vi "Mosbus_Master.vi"() -> ()   [LabVIEW 2020]
uses:
  <vilib>/NI/Modbus Library/API/Wrapper/Create TCP Master.vi
  <vilib>/ErrorRing/Error Ring.xnode
  <vilib>/NI/Modbus Library/API/Master/Modbus Master.lvclass
  <vilib>/NI/Modbus Library/API/Wrapper/API Main.lvlib
panel:
  in  "Thermometer":u16(slide) scale=0.0..100.0
  in  "Array 2":u16[](array[slide]) scale=0.0..100.0
  in  "Boolean 4":bool
  in  "Boolean 3":bool
  in  "Boolean 2":bool
  in  "Boolean":bool
  in  "stop":bool
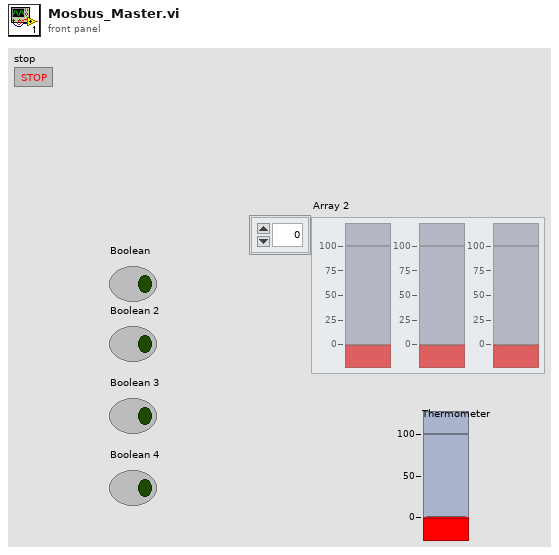
[diagram p1: front panel]
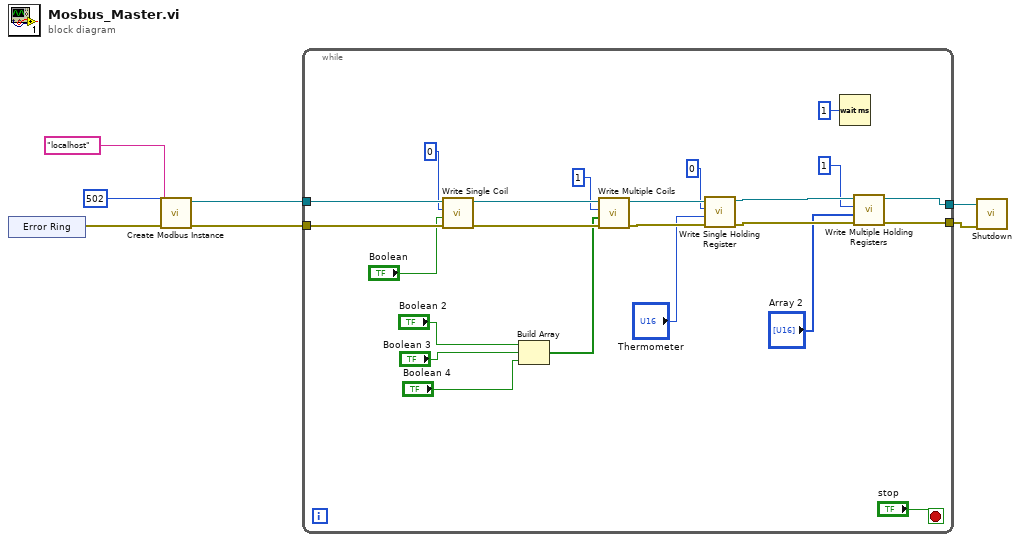
[diagram p0: block diagram]
diagram:
  n1 = xnode "Error Ring"() -> ("error out"=w5:errorcluster)
  n2 = call-poly <vilib>:"Create Modbus Instance.vi"("error in"=w5, "port (502)"=u16 502, "address"="localhost") -> ("error out"=w3:errorcluster, "TCP master instance"=w4:refnum<class "Modbus Master.lvclass">)  [unwired: 7 in]
  n3 = while {
    tunnel: w4 -> [w29]
    tunnel: w3 -> [w28]
    tunnel: [w13] -> w2
    tunnel: [w12] -> w1
    stop <- "stop" stop-if-true
    n4 = call-dynamic "Write Single Coil.vi"("error in"=w28, "coil to write"="Boolean", "address"=u16 0, "Modbus master in"=w29) -> ("error out"=w21:errorcluster, "Modbus master out"=w22:refnum<class "Modbus Master.lvclass">)  [unwired: 6 in]
    n5 = Build Array("Boolean 2", "Boolean 3", "Boolean 4") -> (w20:bool[])
    n6 = call-dynamic "Write Multiple Coils.vi"("error in"=w21, "coils to write"=w20, "starting address"=u16 1, "Modbus master in"=w22) -> ("error out"=w16:errorcluster, "Modbus master out"=w17:refnum<class "Modbus Master.lvclass">)  [unwired: 6 in]
    n7 = call-dynamic "Write Single Holding Register.vi"("error in"=w16, "register to write"="Thermometer", "address"=u16 0, "Modbus master in"=w17) -> ("error out"=w14:errorcluster, "Modbus master out"=w15:refnum<class "Modbus Master.lvclass">)  [unwired: 6 in]
    n8 = Wait (ms)(milliseconds to wait=u32 1) -> ()  [unwired: 1 out]
    n9 = call-dynamic "Write Multiple Holding Registers.vi"("error in"=w14, "registers to write"="Array 2", "starting address"=u16 1, "Modbus master in"=w15) -> ("error out"=w12:errorcluster, "Modbus master out"=w13:refnum<class "Modbus Master.lvclass">)  [unwired: 6 in]
  }
  n10 = call-dynamic "Shutdown.vi"("error in"=w1, "Modbus master in"=w2) -> ()  [unwired: 9 in, 1 out]
